vi "停止报文.vi"() -> ()   [LabVIEW 2023]
panel:
  out "最终输出报文":string
  # "90是停止 12\n18是使能 3 \n20是通信类型4"
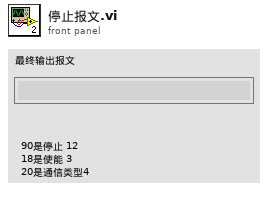
[diagram p1: front panel]
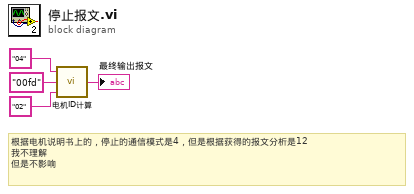
[diagram p0: block diagram]
diagram:
  # "根据电机说明书上的，停止的通信模式是4，但是根据获得的报文分析是12\n我不理解\n但是不影响"
  n1 = call "电机ID计算.vi"("电机ID"="02", "主机id"="00fd", "通信模式"="04") -> ("最终输出报文"=→"最终输出报文":string)
